vi "MultiChannnel_With_Origin.vi"() -> ()   [LabVIEW 2024]
uses:
  <vilib>/DAQmx/read.llb/DAQmx Read (Analog 1D Wfm NChan NSamp).vi
  <vilib>/DAQmx/create/channels.llb/DAQmx Create Channel (AI-Voltage-Basic).vi
  <vilib>/DAQmx/configure/timing.llb/DAQmx Timing (Sample Clock).vi
  <vilib>/DAQmx/miscellaneous.llb/DAQmx Fill In Error Info.vi
  <vilib>/Waveform/WDTOps.llb/WDT Index Channel DBL.vi
panel:
  in  "stop":bool
  out "Numeric":i32
  out "element 3":dbl
  out "element 2":dbl
  out "element":dbl
  out "appended array":dbl[][](array[numeric])
  out "Y 3":dbl[](array[numeric])
  out "Y 2":dbl[](array[numeric])
  out "Y":dbl[](array[numeric])
  in  "Get Orogin":bool
  out "Waveform Graph":waveform(dbl)[](graph)
  in  "samples per channel":i32=500
  in  "sample mode":i32(ring)=10123 items=["Continuous Samples"=10123, "Finite Samples"=10178, "Hardware Timed Single Point"=12522]
  in  "rate":dbl=1000.0 format="%0.2f"
  in  "physical channels":tag="Dev2/ai0:2"
  # "Phy Channel -> Set to 0-2\nRate 1000Hz\nSampleMode  -> Contenious Sampling\nSample per Channel -> 100"
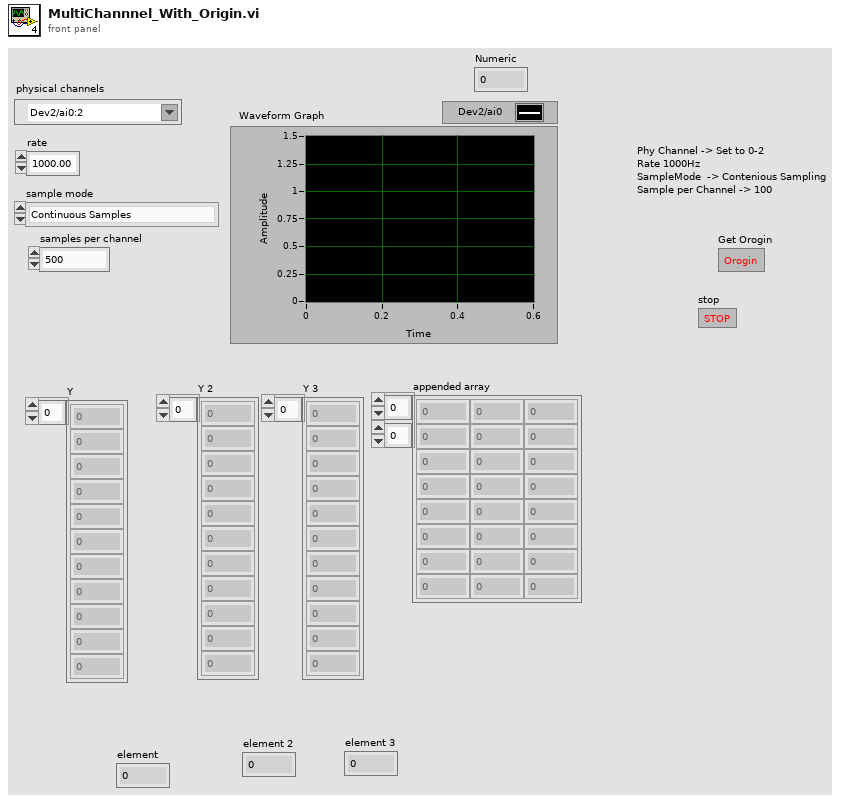
[diagram p1: front panel]
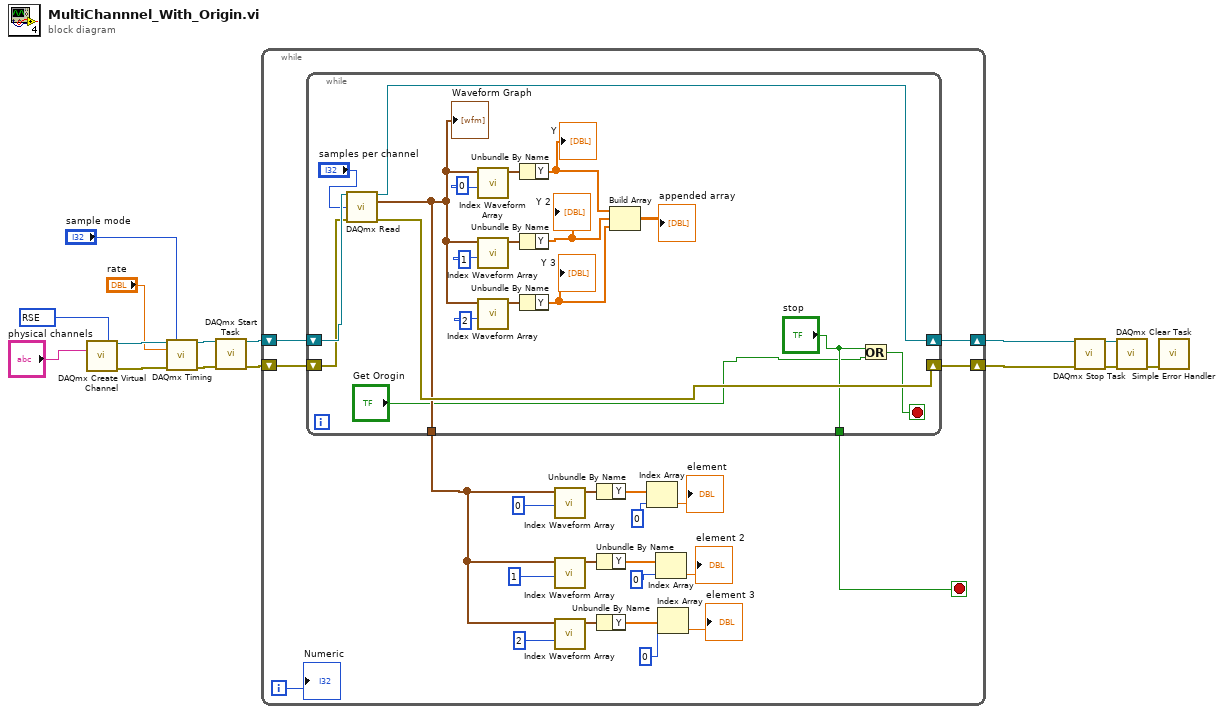
[diagram p0: block diagram]
diagram:
  w1 = 10083 items=["Default"=-1, "RSE"=10083, "NRSE"=10078, "Differential"=10106, "Pseudodifferential"=12529] ("input terminal configuration")
  n1 = call-poly <vilib>:"DAQmx Create Virtual Channel.vi"("input terminal configuration"=w1, "physical channels"="physical channels") -> ("task out"=w7:refnum<k21>, "error out"=w6:errorcluster)  [unwired: 12 in]
  n2 = call-poly <vilib>:"DAQmx Timing.vi"("task/channels in"=w7, "sample mode"="sample mode", "rate"="rate", "error in"=w6) -> ("task out"=w5:refnum<k21>, "error out"=w4:errorcluster)  [unwired: 10 in]
  n3 = call <vilib>:"DAQmx Start Task.vi"("task/channels in"=w5, "error in"=w4) -> ("task out"=w14:refnum<k21>, "error out"=w13:errorcluster)  [unwired: 12 in]
  n4 = while {
    shift-right: [w34] -> w11
    shift-left: w14 -> [w37]
    shift-right: [w35] -> w12
    shift-left: w13 -> [w36]
    i -> [w20]
    stop <- w16 stop-if-true
    n5 = while {
      shift-right: [w53] -> w34
      shift-left: w37 -> [w56]
      shift-right: [w54] -> w35
      shift-left: w36 -> [w55]
      tunnel: [w41] -> w30
      tunnel: ["stop"] -> w16
      stop <- w40 stop-if-true
      n6 = call-poly <vilib>:"DAQmx Read.vi"("task/channels in"=w56, "number of samples per channel"="samples per channel", "error in"=w55) -> ("task out"=w53:refnum<k21>, "data"=w41:waveform(dbl)[], "error out"=w54:errorcluster)  [unwired: 10 in]
      "Waveform Graph" <- w41
      n7 = call-poly <vilib>:"Index Waveform Array.vi"("index"=0, "waveform array"=w41) -> ("waveform"=w50:waveform(dbl))  [unwired: 8 in, 1 out]
      n8 = call-poly <vilib>:"Index Waveform Array.vi"("index"=1, "waveform array"=w41) -> ("waveform"=w48:waveform(dbl))  [unwired: 8 in, 1 out]
      n9 = call-poly <vilib>:"Index Waveform Array.vi"("index"=2, "waveform array"=w41) -> ("waveform"=w46:waveform(dbl))  [unwired: 8 in, 1 out]
      n10 = Unbundle By Name(w50) -> ("Y"=w45:dbl[])
      "Y" <- w45
      n11 = Unbundle By Name(w48) -> ("Y"=w44:dbl[])
      "Y 2" <- w44
      n12 = Unbundle By Name(w46) -> ("Y"=w43:dbl[])
      "Y 3" <- w43
      n13 = Build Array(w45, w44, w43) -> (→"appended array":dbl[][])
      n14 = Or(x="stop", y="Get Orogin") -> (x .or. y?=w40:bool)
    }
    n15 = call-poly <vilib>:"Index Waveform Array.vi"("index"=0, "waveform array"=w30) -> ("waveform"=w33:waveform(dbl))  [unwired: 8 in, 1 out]
    n16 = call-poly <vilib>:"Index Waveform Array.vi"("index"=1, "waveform array"=w30) -> ("waveform"=w32:waveform(dbl))  [unwired: 8 in, 1 out]
    n17 = call-poly <vilib>:"Index Waveform Array.vi"("index"=2, "waveform array"=w30) -> ("waveform"=w31:waveform(dbl))  [unwired: 8 in, 1 out]
    n18 = Unbundle By Name(w33) -> ("Y"=w29:dbl[])
    n19 = Unbundle By Name(w32) -> ("Y"=w24:dbl[])
    n20 = Unbundle By Name(w31) -> ("Y"=w25:dbl[])
    n21 = Index Array(array=w29, index=0) -> (element=→"element":dbl)
    n22 = Index Array(array=w24, index=0) -> (element=→"element 2":dbl)
    n23 = Index Array(array=w25, index=0) -> (element=→"element 3":dbl)
    "Numeric" <- w20
  }
  n24 = call <vilib>:"DAQmx Stop Task.vi"("task/channels in"=w11, "error in"=w12) -> ("task out"=w9:refnum<k21>, "error out"=w10:errorcluster)  [unwired: 12 in]
  n25 = call <vilib>:"DAQmx Clear Task.vi"("task in"=w9, "error in"=w10) -> ("error out"=w8:errorcluster)  [unwired: 13 in]
  n26 = call <vilib>:"Simple Error Handler.vi"("error in (no error)"=w8) -> ()  [unwired: 4 in, 5 out]
